vi "json path array to path.vi"(1 "path":string[](array[string])) -> (0 "String":string)   [LabVIEW 2016, in "JSON Document.lvclass"]
uses:
  JSON Document.lvclass
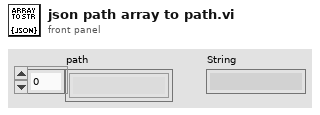
[diagram p1: front panel]
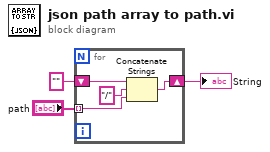
[diagram p0: block diagram]
diagram:
  n1 = for {
    tunnel: "path" -> [w6] mode=indexing
    shift-right: [w4] -> w1
    shift-left: "" -> [w7]
    n2 = Concatenate Strings(w7, "/" ("string"), w6) -> (w4:string)
  }
  "String" <- w1
